vi "Read All FP Properties.vi"(8 "error in (no error)":errorcluster, 9 "Read":bool, 11 "VI in":refnum<vi>) -> (0 "error out":errorcluster, 3 "Properties out":T1)   [LabVIEW 2020]
uses:
  TDefs/FP Items Properties.ctl
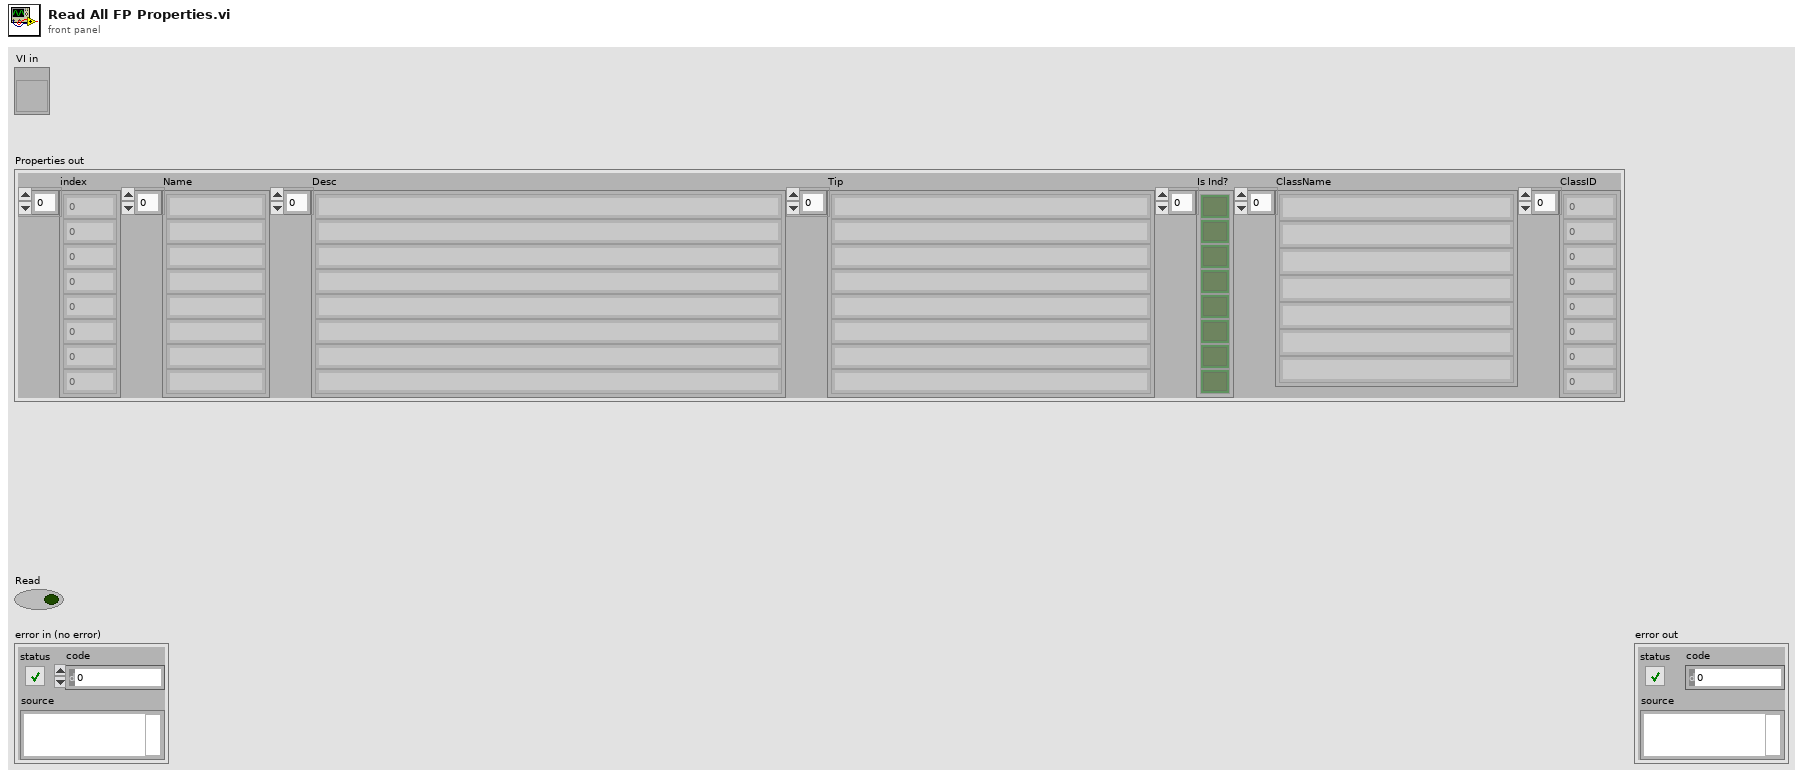
[diagram p1: front panel]
types:
  T1 = typedef "FP Items Properties.ctl" = cluster{"index":i32[], "Name":string[], "Desc":string[], "Tip":string[], "Is Ind?":bool[], "ClassName":string[], "ClassID":u32[]}
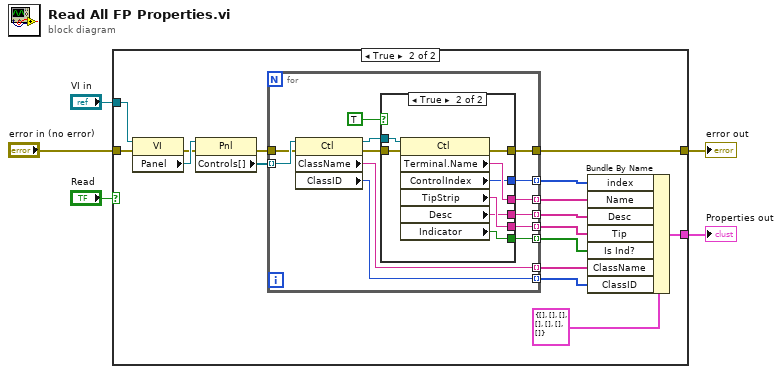
[diagram p0: block diagram]
diagram:
  n1 = case shown="True" "Read" {
    tunnel: "VI in" -> [_ w22]
    tunnel: [w6 w17] -> w1
    tunnel: "error in (no error)" -> [w6 w16]
    tunnel: [_ w15] -> w5
    frame False {
    }
    frame True {
      n2 = property class="VI"(reference=w22, error in=w16) -> (error out=w18:errorcluster, "Panel"=w21:refnum<vi>)  [unwired: 1 out]
      n3 = property class="Pnl"(reference=w21, error in=w18) -> (error out=w19:errorcluster, "Controls[]"=w20:refnum<vi>[])  [unwired: 1 out]
      n4 = for {
        tunnel: w20 -> [w35] mode=indexing
        tunnel: [w33] -> w8 mode=indexing
        tunnel: [w34] -> w9 mode=indexing
        tunnel: [w31] -> w14 mode=indexing
        tunnel: [w30] -> w13 mode=indexing
        tunnel: [w29] -> w11 mode=indexing
        tunnel: [w28] -> w12 mode=indexing
        tunnel: [w26] -> w10 mode=indexing
        tunnel: w19 -> [w25]
        tunnel: [w23] -> w17
        n5 = property class="Ctl"(reference=w35, error in=w25) -> (reference out=w32:refnum<vi>, error out=w24:errorcluster, "ClassName"=w33:string, "ClassID"=w34:u32)
        n6 = case shown="True" TRUE {
          tunnel: w32 -> [_ w43]
          tunnel: [_ w38] -> w31
          tunnel: [_ w42] -> w30
          tunnel: [_ w41] -> w29
          tunnel: [_ w40] -> w28
          tunnel: [_ w39] -> w26
          tunnel: w24 -> [_ w37]
          tunnel: [_ w36] -> w23
          frame False {
          }
          frame True {
            n7 = property class="Ctl"(reference=w43, error in=w37) -> (error out=w36:errorcluster, "Terminal.Name"=w42:string, "ControlIndex"=w38:i32, "TipStrip"=w41:string, "Desc"=w40:string, "Indicator"=w39:bool)  [unwired: 1 out]
          }
        }
      }
      n8 = Bundle By Name(cluster=T1 {"index"=[], "Name"=[], "Desc"=[], "Tip"=[], "Is Ind?"=[], "ClassName"=[], "ClassID"=[]} ("Properties in"), "index"=w14, "Name"=w13, "Desc"=w12, "Tip"=w11, "Is Ind?"=w10, "ClassName"=w8, "ClassID"=w9) -> (w15:T1)
    }
  }
  "Properties out" <- w5
  "error out" <- w1
